vi "open color cam.vi"() -> ()   [LabVIEW 2015]
uses:
  <vilib>/vision/NI_Vision_Development_Module.lvlib
panel:
  out "error out 2":errorcluster
  out "error out":errorcluster
  out "Image Out":T1(plugin-control)
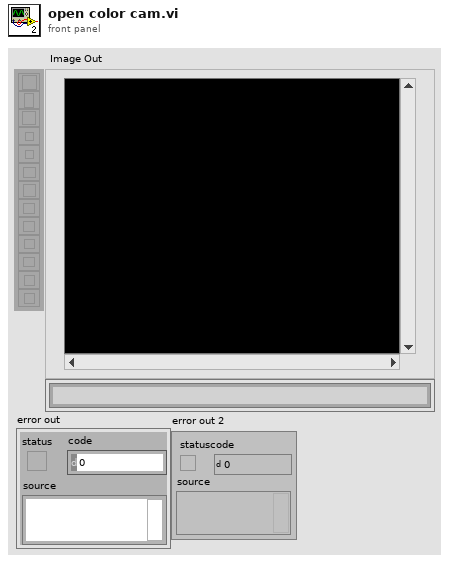
[diagram p1: front panel]
types:
  T1 = typedef "IMAQ Image.ctl" = refnum<image>
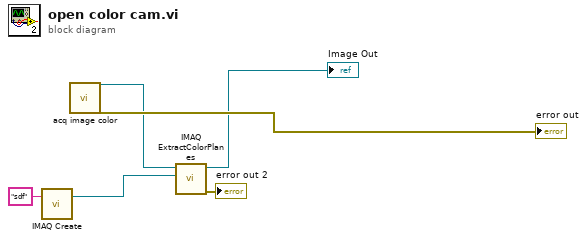
[diagram p0: block diagram]
diagram:
  n1 = call "IMAQ Create"("Image Name"="sdf") -> ("New Image"=w2:T1)  [unwired: 4 in, 1 out]
  n2 = call "acq image color.vi"() -> ("Image Out"=w5:T1, "error out"=→"error out":errorcluster)  [unwired: 26 in]
  n3 = call "IMAQ ExtractColorPlanes"("Red or Hue Plane"=w2, "Image Src"=w5) -> ("error out"=→"error out 2":errorcluster, "Red or Hue Plane out"=→"Image Out":T1)  [unwired: 6 in, 2 out]
